vi "GEOM_GetHdrType.vi"(10 "arg in":string) -> (1 "type":string, 2 "arg out":string)   [LabVIEW 2016]
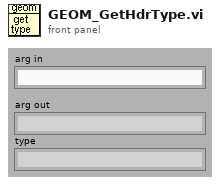
[diagram p1: front panel]
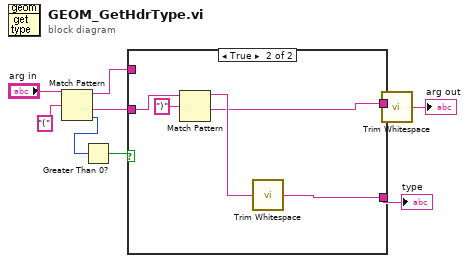
[diagram p0: block diagram]
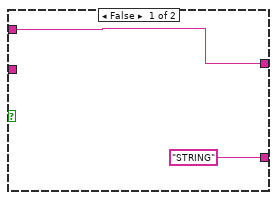
[diagram p2: hidden frame]
diagram:
  n1 = Match Pattern(string="arg in", regular expression="(") -> (before substring=w4:string, after substring=w5:string, offset past match=w7:i32)  [unwired: 2 out]
  n2 = Greater Than 0?(x=w7) -> (x > 0?=w6:bool)
  n3 = case shown="True" w6 {
    tunnel: w5 -> [_ w16]
    tunnel: w4 -> [w10 _]
    tunnel: [w10 w12] -> w3
    tunnel: ["STRING" ("trimmed string") w13] -> w2
    frame False {
    }
    frame True {
      n4 = Match Pattern(string=w16, regular expression=")") -> (before substring=w14:string, after substring=w12:string)  [unwired: 3 out]
      n5 = call <vilib>:"Trim Whitespace.vi"("string"=w14) -> ("trimmed string"=w13:string)  [unwired: 1 in]
    }
  }
  "type" <- w2
  n6 = call <vilib>:"Trim Whitespace.vi"("string"=w3) -> ("trimmed string"=→"arg out":string)  [unwired: 1 in]
